vi "Execute Command.vi"(8 "error in (no error)":errorcluster, 10 "Resize Menu in":refnum<class "Resize Menu.lvclass">, 11 "User Interface References":T1={"This VI"=refnum, "User Interace Plugin"=refnum, "UI Picture Container References"={"Header Image"=refnum, "Footer Image"=refnum}, "Sliding Menu XControl"=refnum, "Menu Container"=refnum, "UI Configuration Information"={"Space Between Buttons"=3, "Number of Buttons to Show"=6, "Header Image"=path "Images/Blue Background.bmp", "Footer Image"=path "Images/Blue Background.bmp"}, "Header Text"=refnum}) -> (0 "error out":errorcluster, 1 "Stop?":bool, 2 "Resize Menu out":refnum<class "Resize Menu.lvclass">, 3 "User Interface References Out":T1={"This VI"=refnum, "User Interace Plugin"=refnum, "UI Picture Container References"={"Header Image"=refnum, "Footer Image"=refnum}, "Sliding Menu XControl"=refnum, "Menu Container"=refnum, "UI Configuration Information"={"Space Between Buttons"=3, "Number of Buttons to Show"=6, "Header Image"=path "Images/Blue Background.bmp", "Footer Image"=path "Images/Blue Background.bmp"}, "Header Text"=refnum})   [LabVIEW 2011, in "Resize Menu.lvclass"]
uses:
  Resize Menu.lvclass
  Main Type Definitions/User Interface Type Definitions.ctl
  Main Type Definitions/UI Picture Containers.ctl
  Sliding Menu/Sliding Menu Library/Sliding Menu xControl/Sliding Menu XControl.xctl
  UI Control Definitions/UI Configuration Information.ctl
  UI Command Manager.lvclass
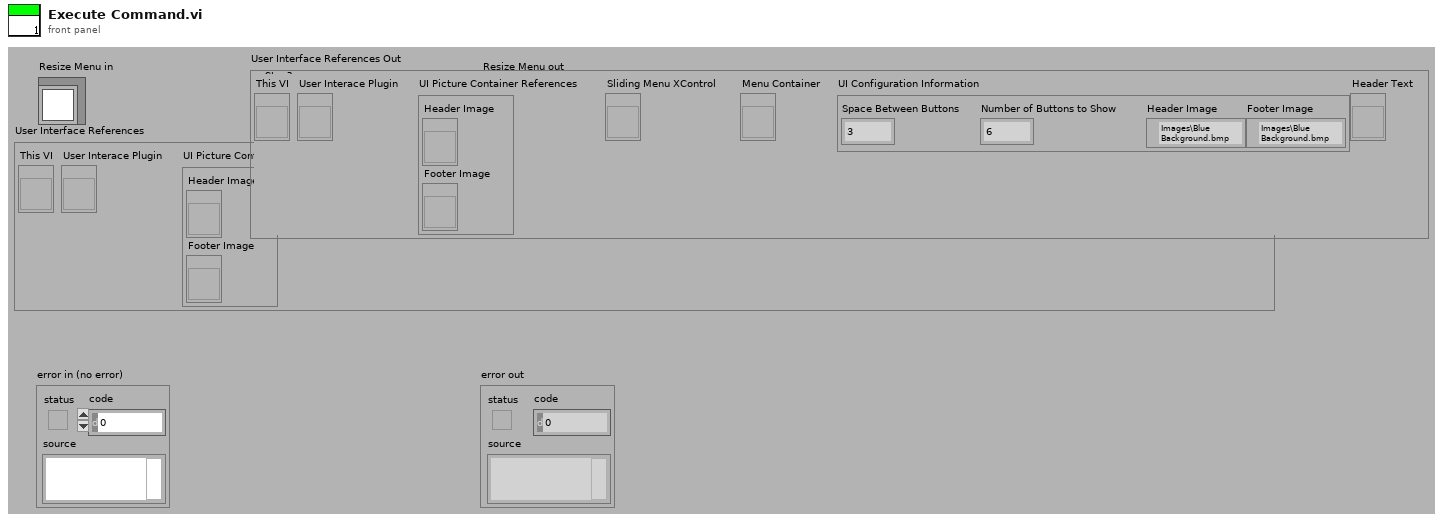
[diagram p1: front panel]
types:
  T1 = typedef "User Interface Type Definitions.ctl" = cluster{"This VI":refnum<vi>, "User Interace Plugin":refnum<vi>, "UI Picture Container References":T2, "Sliding Menu XControl":refnum<vi>, "Menu Container":refnum<vi>, "UI Configuration Information":T3, "Header Text":refnum<vi>}
  T2 = typedef "UI Picture Containers.ctl" = cluster{"Header Image":refnum<vi>, "Footer Image":refnum<vi>}
  T3 = typedef "UI Configuration Information.ctl" = cluster{"Space Between Buttons":i32, "Number of Buttons to Show":i32, "Header Image":path, "Footer Image":path}
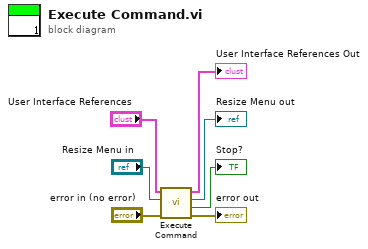
[diagram p0: block diagram]
diagram:
  n1 = call-parent "Execute Command.vi"("error in (no error)"="error in (no error)", "UI Command Manager in"="Resize Menu in", "User Interface References"="User Interface References") -> ("error out"=→"error out":errorcluster, "Stop?"=→"Stop?":bool, "UI Command Manager out"=→"Resize Menu out":refnum<class "Resize Menu.lvclass">, "User Interface References Out"=→"User Interface References Out":T1)  [unwired: 5 in]
